vi "Sequence Update Table for Spartan 5.0.vi"(8 "error in (no error)":errorcluster, 11 "Connection Refnum":T1) -> (0 "error out":errorcluster, 3 "Connection Refnum":T1)   [LabVIEW 2011]
uses:
  Summitek EXT/ODBC/SQL Controls/Connection Refnum.ctl
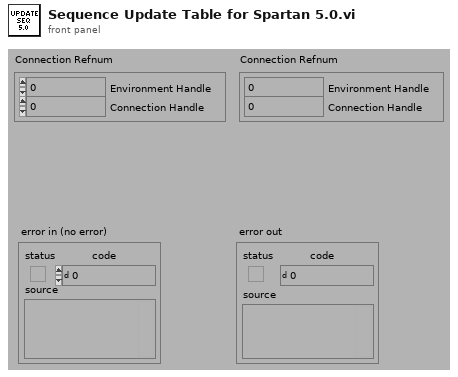
[diagram p1: front panel]
types:
  T1 = typedef "Connection Refnum.ctl" = cluster{"Environment Handle":i32, "Connection Handle":i32}
  T2 = typedef "Statement Refnum.ctl" = cluster{"Statement Handle":i32, "Parameter Number":u16}
  T3 = typedef "Sequence Record.ctl" = cluster{"ixSequence":i32, "sxSequenceId":string, "sDescription":string, "sCreator":string, "tCreationDate":timestamp, "sModifier":string, "tModifiedDate":timestamp, "fApproved":bool, "fSpartanSetsSN":bool, "fOverwriteData":bool, "fStopOnFail":bool, "fDisableQuickMode":bool, "fPartialExecution":bool, "fAutoNextItem":bool, "fDoNotPrintOnFail":bool}
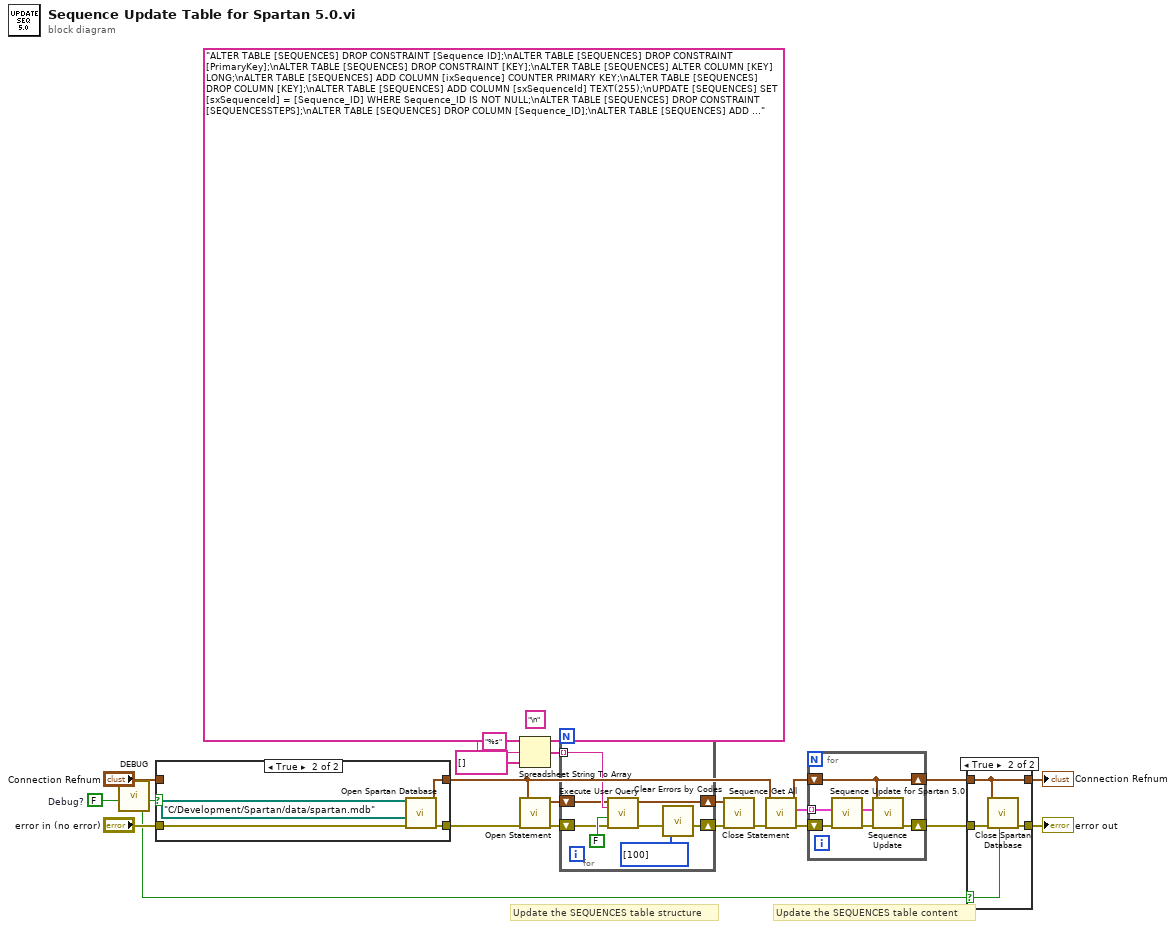
[diagram p0: block diagram]
diagram:
  w3 = FALSE  # Debug?
  # "Update the SEQUENCES table content"
  # "Update the SEQUENCES table structure"
  n1 = call "DEBUG.vi"("Dev DEBUG? (f)"=w3) -> ("DEBUG?"=w2:bool)  [unwired: 1 in, 5 out]
  n2 = case shown="True" w2 {
    tunnel: "Connection Refnum" -> [w25 _]
    tunnel: "error in (no error)" -> [w24 w28]
    tunnel: [w24 w27] -> w5
    tunnel: [w25 w26] -> w4
    frame False {
    }
    frame True {
      (unwired) path "C:/Development/Spartan/data/spartan.mdb" ("DB Path")
      n3 = call "Open Spartan Database.vi"("error in (no error)"=w28) -> ("error out"=w27:errorcluster, "Connection Refnum"=w26:T1)  [unwired: 2 in, 7 out]
    }
  }
  n4 = Spreadsheet String To Array(delimiter (Tab)="\n", format string="%s", spreadsheet string="ALTER TABLE [SEQUENCES] DROP CONSTRAINT [Sequence ID];\nALTER TABLE [SEQUENCES] DROP CONSTRAINT [PrimaryKey];\nALTER TABLE [SEQUENCES] DROP CONSTRAINT [KEY];\nALTER TABLE [SEQUENCES] ALTER COLUMN [KEY] LONG;\nALTER TABLE [SEQUENCES] ADD COLUMN [ixSequence] COUNTER PRIMARY KEY;\nALTER TABLE [SEQUENCES] DROP COLUMN [KEY];\nALTER TABLE [SEQUENCES] ADD COLUMN [sxSequenceId] TEXT(255);\nUPDATE [SEQUENCES] SET [sxSequenceId] = [Sequence_ID] WHERE Sequence_ID IS NOT NULL;\nALTER TABLE [SEQUENCES] DROP CONSTRAINT [SEQUENCESSTEPS];\nALTER TABLE [SEQUENCES] DROP COLUMN [Sequence_ID];\nALTER TABLE [SEQUENCES] ADD COLUMN [sDescription] TEXT(255);\nUPDATE [SEQUENCES] SET [sDescription] = [Description];\nALTER TABLE [SEQUENCES] DROP COLUMN [Description]; \nALTER TABLE [SEQUENCES] ADD COLUMN [sCreator] TEXT(255);\nUPDATE [SEQUENCES] SET [sCreator] = [Creator];\nALTER TABLE [SEQUENCES] DROP COLUMN [Creator];\nALTER TABLE [SEQUENCES] ADD COLUMN [tCreationDate] DATE;\nALTER TABLE [SEQUENCES] ADD COLUMN [sTemp1] TEXT(255);\nUPDATE [SEQUENCES] SET [sTemp1] = [Creation_Date];\nALTER TABLE [SEQUENCES] DROP COLUMN [Creation_Date];\nALTER TABLE [SEQUENCES] ADD COLUMN [sModifier] TEXT(255);\nUPDATE [SEQUENCES] SET [sModifier] = [Modifier];\nALTER TABLE [SEQUENCES] DROP COLUMN [Modifier];\nALTER TABLE [SEQUENCES] ADD COLUMN [tModifiedDate] DATE;\nALTER TABLE [SEQUENCES] ADD COLUMN [sTemp2] TEXT(255);\nUPDATE [SEQUENCES] SET [sTemp2] = [Modified_Date];\nALTER TABLE [SEQUENCES] DROP COLUMN [Modified_Date];\nALTER TABLE [SEQUENCES] ADD COLUMN [fApproved] LONG;\nALTER TABLE [SEQUENCES] ADD COLUMN [fSpartanSetsSN] LONG;\nALTER TABLE [SEQUENCES] ADD COLUMN [fOverwriteData] LONG;\nALTER TABLE [SEQUENCES] ADD COLUMN [fStopOnFail] LONG;\nALTER TABLE [SEQUENCES] ADD COLUMN [fDisableQuickMode] LONG;\nALTER TABLE [SEQUENCES] ADD COLUMN [fPartialExecution] LONG;\nALTER TABLE [SEQUENCES] ADD COLUMN [fAutoNextItem] LONG;\nALTER TABLE [SEQUENCES] ADD COLUMN [sTemp3] TEXT(255);\nUPDATE [SEQUENCES] SET [sTemp3] = [Product_Identifier];\nALTER TABLE [SEQUENCES] DROP COLUMN [Product_Identifier];\nALTER TABLE [SEQUENCES] ADD COLUMN [sTemp4] TEXT(255);\nUPDATE [SEQUENCES] SET [sTemp4] = [Settings];\nALTER TABLE [SEQUENCES] DROP COLUMN [Settings];\nUPDATE [SEQUENCES] SET [sCreator] = [sCreator]+'-'+[sTemp1]+'-'+[sTemp2]+'-'+[sTemp3]+'-'+[sTemp4];\nALTER TABLE [SEQUENCES] DROP COLUMN [sTemp1];\nALTER TABLE [SEQUENCES] DROP COLUMN [sTemp2];\nALTER TABLE [SEQUENCES] DROP COLUMN [sTemp3];\nALTER TABLE [SEQUENCES] DROP COLUMN [sTemp4];\nALTER TABLE [SEQUENCES] DROP COLUMN [PDA];" ("User Query"), array type (2D Dbl)=string[] []) -> (array=w22:string[])
  n5 = call "Open Statement.vi"("error in (no error)"=w5, "Connection Refnum"=w4) -> ("error out"=w17:errorcluster, "Statement Refnum"=w16:T2)  [unwired: 4 out]
  n6 = for {
    shift-right: [w29] -> w15
    shift-left: w17 -> [w33]
    tunnel: w22 -> [w35] mode=indexing
    shift-right: [w32] -> w14
    shift-left: w16 -> [w34]
    n7 = call "Execute User Query.vi"("error in (no error)"=w33, "Return Data? (f)"=FALSE, "User Query"=w35, "Statement Refnum"=w34) -> ("error out"=w30:errorcluster, "Statement Refnum"=w32:T2)  [unwired: 2 out]
    n8 = call "Clear Errors by Codes.vi"("Error Codes\nto Clear (Empty)"=i32[] [100] ("Error Codes\nto Clear (Empty)"), "error in (no error)"=w30) -> ("error out"=w29:errorcluster)  [unwired: 5 out]
  }
  n9 = call "Close Statement.vi"("error in (no error)"=w15, "Statement Refnum"=w14) -> ("error out"=w13:errorcluster)  [unwired: 5 out]
  n10 = call "Sequence Get All.vi"("error in (no error)"=w13, "Connection Refnum"=w4) -> ("error out"=w12:errorcluster, "Sequence Records"=w19:T3[], "Connection Refnum"=w18:T1)  [unwired: 2 in, 5 out]
  n11 = for {
    shift-right: [w42] -> w11
    shift-left: w12 -> [w40]
    shift-right: [w41] -> w10
    shift-left: w18 -> [w41]
    tunnel: w19 -> [w37] mode=indexing
    n12 = call "Sequence Update for Spartan 5.0.vi"("error in (no error)"=w40, "Old Sequence Record"=w37) -> ("error out"=w39:errorcluster, "New Sequence Record"=w38:T3)  [unwired: 8 out]
    n13 = call "Sequence Update.vi"("error in (no error)"=w39, "Sequence Record"=w38, "Connection Refnum"=w41) -> ("error out"=w42:errorcluster)  [unwired: 8 out]
  }
  n14 = case shown="True" w2 {
    selector: w2 -> [_ w45]
    tunnel: w11 -> [w44 w48]
    tunnel: w10 -> [w43 w46]
    tunnel: [w43 w46] -> w9
    tunnel: [w44 w47] -> w8
    frame False {
    }
    frame True {
      n15 = call "Close Spartan Database.vi"("Force Close? (f)"=w45, "error in (no error)"=w48, "Connection Refnum"=w46) -> ("error out"=w47:errorcluster)  [unwired: 2 in, 6 out]
    }
  }
  "error out" <- w8
  "Connection Refnum" <- w9
